vi "Initialize.vi"(6 "iName":string, 7 "iType":string, 8 "error in (no error)":errorcluster, 11 "Application Data":path) -> (0 "error out":errorcluster, 3 "Assembler out":refnum<class "Assembler.lvclass">)   [LabVIEW 2016, in "CLD Exam - ATM.lvlib" / "Assembler.lvclass"]
uses:
  Assembler.lvclass
  Log/Application Log/Log Level.ctl
  Log/Text File Sink/Configuration.ctl
  Log/Application Log/Application Log.lvclass
  Assembler.lvclass/Assembler.ctl
  Log/Text File Sink/Text File Sink.lvclass
  D:/Repos/Stream/software/Log/Log Sink/Log Sink.lvclass
  Mediator/Classes/Message Broker Interface Ref/Message Broker Interface Ref.lvclass
  Log/Global Application Log/Global Application Log.lvclass
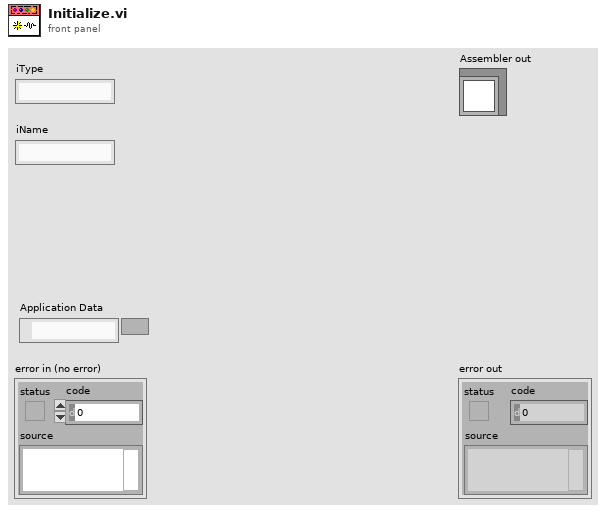
[diagram p1: front panel]
types:
  T1 = typedef "Stream Log.lvlib/Text File Sink.lvclass/Configuration.ctl" = cluster{"Folder":path, "Name":string, "Extension":string, "Mangle":bool, "Append":bool, "Flush":bool, "Max Size (MB)":i64, "Timestamp Filename":bool}
  T2 = typedef "Stream Log.lvlib/Application Log.lvclass/Log Level.ctl" = enum16{"Imperative", "Major", "Minor", "Debug", "Off"}
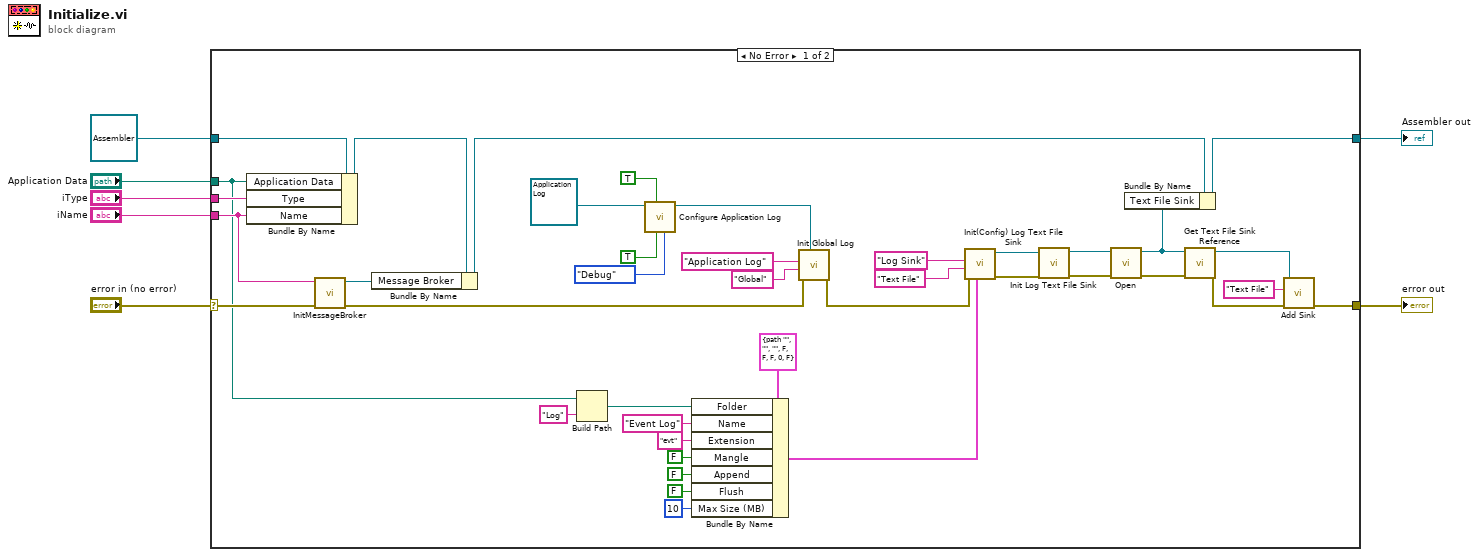
[diagram p0: block diagram]
diagram:
  n1 = case shown="No Error" "error in (no error)" {
    selector: "error in (no error)" -> [w45 w49]
    tunnel: [w23 w49] -> w6
    tunnel: [w21 w48] -> w4
    tunnel: refnum<class "Assembler.lvclass"> refnum ("Assembler in") -> [w46 w48]
    tunnel: "iType" -> [w47 _]
    tunnel: "iName" -> [w44 _]
    tunnel: "Application Data" -> [w9 _]
    frame No Error {
      n2 = Bundle By Name(cluster=w46, "Application Data"=w9, "Type"=w47, "Name"=w44) -> (w43:refnum<class "Assembler.lvclass">)
      n3 = call "InitMessageBroker.vi"("error in (no error)"=w45, "Broker Name"=w44) -> ("error out"=w35:errorcluster, "Message Broker Interface Ref out"=w42:refnum<class "Message Broker Interface Ref.lvclass">)  [unwired: 8 in]
      n4 = Bundle By Name(cluster=w43, "Message Broker"=w42) -> (w22:refnum<class "Assembler.lvclass">)
      n5 = Build Path(base path=w9, name or relative path="Log") -> (appended path=w18:path)
      n6 = call-dynamic "Configure Application Log.vi"("Configuration.Level"=Log_Level."Debug", "Configuration.Enabled"=TRUE, "Configuration.Call Chain"=TRUE, "Application Log in"=refnum<class "Application Log.lvclass"> refnum ("Stream Log.lvlib:Application Log.lvclass")) -> ("Application Log out"=w38:refnum<class "Application Log.lvclass">)  [unwired: 6 in, 1 out]
      n7 = Bundle By Name(cluster=T1 {"Folder"=path "", "Name"="", "Extension"="", "Mangle"=FALSE, "Append"=FALSE, "Flush"=FALSE, "Max Size (MB)"=0, "Timestamp Filename"=FALSE} ("Text File Sink Configuration"), "Folder"=w18, "Name"="Event Log", "Extension"="evt", "Mangle"=FALSE, "Append"=FALSE, "Flush"=FALSE, "Max Size (MB)"=i64 10) -> (w10:T1)
      n8 = call "Init Global Log.vi"("Application Log in"=w38, "error in (no error)"=w35, "iType"="Global", "iName"="Application Log") -> ("error out"=w32:errorcluster)  [unwired: 7 in]
      n9 = call "Init(Config) Log Text File Sink.vi"("Text File Sink Configuration"=w10, "error in (no error)"=w32, "iName"="Text File", "iType"="Log Sink") -> ("error out"=w30:errorcluster, "Text File Sink out"=w31:refnum<class "Text File Sink.lvclass">)  [unwired: 6 in]
      n10 = call "Init Log Text File Sink.vi"("error in (no error)"=w30, "Text File Sink in"=w31) -> ("error out"=w28:errorcluster, "Text File Sink out"=w29:refnum<class "Text File Sink.lvclass">)  [unwired: 8 in]
      n11 = call "Open.vi"("error in (no error)"=w28, "Text File Sink in"=w29) -> ("error out"=w27:errorcluster, "Text File Sink out"=w20:refnum<class "Text File Sink.lvclass">)  [unwired: 8 in]
      n12 = Bundle By Name(cluster=w22, "Text File Sink"=w20) -> (w21:refnum<class "Assembler.lvclass">)
      n13 = call "Get Text File Sink Reference.vi"("error in (no error)"=w27, "Text File Sink in"=w20) -> ("error out"=w26:errorcluster, "Text File Sink Reference"=w25:refnum<data-value>)  [unwired: 8 in]
      n14 = call "Add Sink.vi"("error in (no error)"=w26, "Sink Name"="Text File", "Log Sink Reference"=w25) -> ("error out"=w23:errorcluster)  [unwired: 8 in]
    }
    frame Error {
    }
  }
  "error out" <- w6
  "Assembler out" <- w4
